vi "NT4150_Write_Number.vi"(4 "options":T1={"Send All"=FALSE, "Keep Duplicates"=FALSE, "rate (hz)"=10}, 6 "timestamp":u64, 8 "error in":errorcluster, 9 "value":dbl, 11 "name":string="Number") -> (0 "error out":errorcluster)   [LabVIEW 2023]
doc: "Update the numeric double to the named topic."
uses:
  <vilib>/Rock Robotics/Network Tables/NT PublishOptions.ctl
  <vilib>/Rock Robotics/Network Tables/NT Datatype.ctl
panel:
  in  "description":string="double"
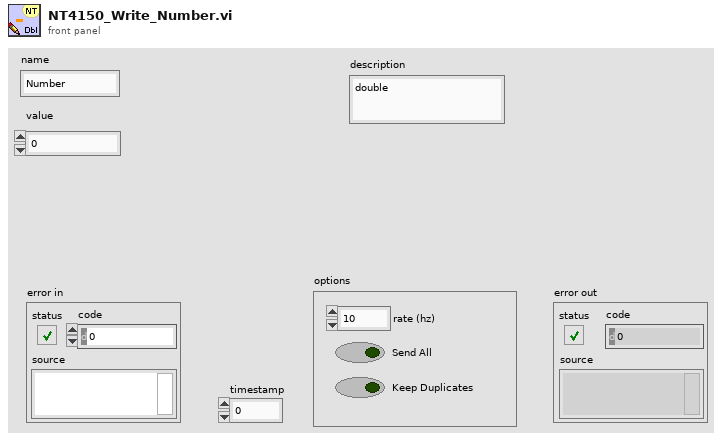
[diagram p1: front panel]
types:
  T1 = typedef "NT PublishOptions.ctl" = cluster{"Send All":bool, "Keep Duplicates":bool, "rate (hz)":u64}
  T2 = typedef "NT Datatype.ctl" = u32
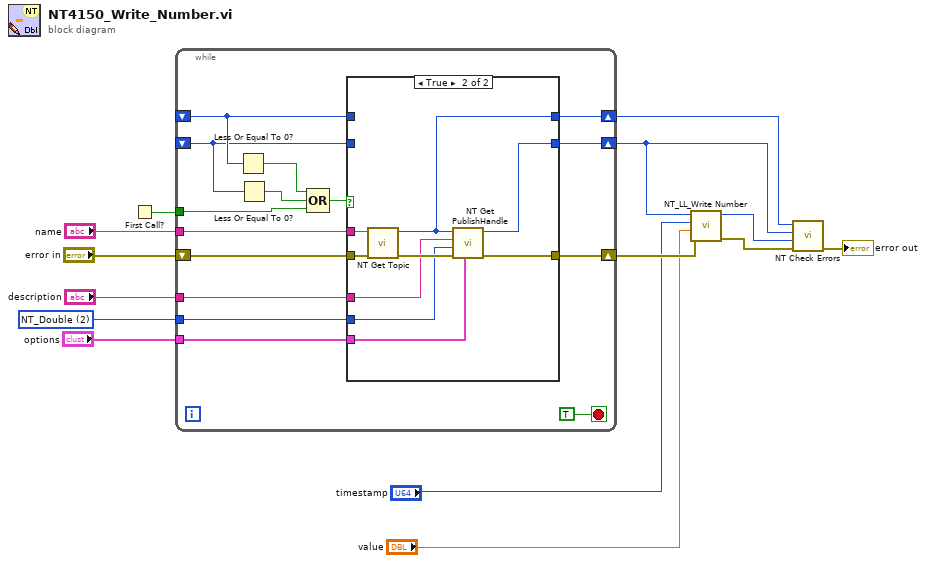
[diagram p0: block diagram]
diagram:
  w12 = T2 2 items=["NT_Unassigned"=0, "NT_Boolean"=1, "NT_Double"=2, "NT_String"=4, "NT_Raw"=8, "NT_BooleanArray"=16, "NT_DoubleArray"=32, "NT_StringArray"=64, "NT_RPC"=128, "NT_Integer"=256, "NT_Float"=512, "NT_IntegerArray"=1024, "NT_FloatArray"=2048] ("NT_Type")
  n1 = First Call?() -> (First Call?: T/F=w1:bool)
  n2 = while {
    tunnel: "name" -> [w28]
    tunnel: w12 -> [w27]
    tunnel: "description" -> [w25]
    tunnel: "options" -> [w24]
    shift-right: [w26] -> w11
    shift-left: "error in" -> [w29]
    shift-right: [w23] -> w5
    shift-left: _ -> [w20]
    shift-right: [w22] -> w3
    shift-left: _ -> [w19]
    tunnel: w1 -> [w16]
    stop <- TRUE stop-if-true
    n3 = Less Or Equal To 0?(x=w20) -> (x <= 0?=w18:bool)
    n4 = Less Or Equal To 0?(x=w19) -> (x <= 0?=w17:bool)
    n5 = Compound Arithmetic op=OR(w18, w17, w16) -> (w15:bool)
    n6 = case shown="True" w15 {
      tunnel: w29 -> [w30 w41]
      tunnel: w28 -> [_ w40]
      tunnel: w27 -> [_ w38]
      tunnel: [w30 w37] -> w26
      tunnel: w25 -> [_ w36]
      tunnel: w24 -> [_ w35]
      tunnel: [w32 w34] -> w23
      tunnel: [w31 w33] -> w22
      tunnel: w20 -> [w32 _]
      tunnel: w19 -> [w31 _]
      frame False {
      }
      frame True {
        n7 = call <vilib>:"NT Get Topic.vi"("error in (no error)"=w41, "name"=w40) -> ("error out"=w39:errorcluster, "topicHandle"=w34:u32)  [unwired: 8 in]
        n8 = call <vilib>:"NT Get PublishHandle.vi"("options"=w35, "error in (no error)"=w39, "NT_Type"=w38, "description"=w36, "topicHandle"=w34) -> ("error out"=w37:errorcluster, "publishHandle"=w33:u32)  [unwired: 5 in]
      }
    }
  }
  n9 = call <vilib>:"NT_LL_Write Number.vi"("error in (no error)"=w11, "value"="value", "timestamp"="timestamp", "publishHandle"=w3) -> ("error out"=w8:errorcluster, "success"=w4:u32)  [unwired: 6 in]
  n10 = call <vilib>:"NT Check Errors.vi"("error in (no error)"=w8, "success"=w4, "pubSubHandle"=w3, "topicHandle"=w5) -> ("error out"=→"error out":errorcluster)  [unwired: 7 in]
